vi "RichToFlatrfcontrol_GetGPSLastLocInfoResponse.vi"(5 "OutputClusterType":T1, 11 "InputCluster":T2) -> (3 "OutputCluster":T1)   [LabVIEW 2024, in "FlexSDR_gRPC_client.lvlib"]
uses:
  rfcontrol_GetGPSLastLocInfoResponse.ctl
  rfcontrol_GetGPSLastLocInfoResponse_Flat.ctl
  FlexSDR_gRPC_client.lvlib
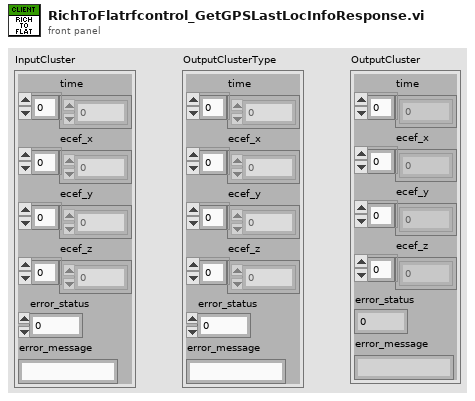
[diagram p1: front panel]
types:
  T1 = typedef "FlexSDR_gRPC_client.lvlib/rfcontrol_GetGPSLastLocInfoResponse_Flat.ctl" = cluster{"time":dbl[], "ecef_x":dbl[], "ecef_y":dbl[], "ecef_z":dbl[], "error_status":i32, "error_message":string}
  T2 = typedef "FlexSDR_gRPC_client.lvlib/rfcontrol_GetGPSLastLocInfoResponse.ctl" = cluster{"time":dbl[], "ecef_x":dbl[], "ecef_y":dbl[], "ecef_z":dbl[], "error_status":i32, "error_message":string}
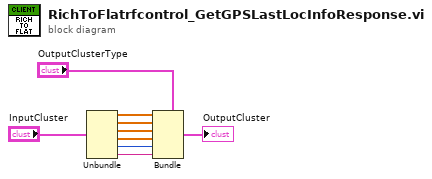
[diagram p0: block diagram]
diagram:
  n1 = Unbundle "Unbundle"("InputCluster") -> ("time"=w6:dbl[], "ecef_x"=w5:dbl[], "ecef_y"=w4:dbl[], "ecef_z"=w3:dbl[], "error_status"=w2:i32, "error_message"=w1:string)
  n2 = Bundle "Bundle"(cluster="OutputClusterType", "time"=w6, "ecef_x"=w5, "ecef_y"=w4, "ecef_z"=w3, "error_status"=w2, "error_message"=w1) -> (→"OutputCluster":T1)
